vi "WLAN Configure SEM.vi"(0 "Instrument Handle In":refnum<k21>, 1 "Selector String":string, 5 "WLAN SEM Configuration":T1={"Sweep Time Auto"=1, "Sweep Time (s)"=0.001, "Span Auto"=1, "Span (Hz)"=100000000.0, "Averaging Enabled"=0, "Averaging Count"=5, "Averaging Type"=0} {"Averaging Type" items=["RMS", "Log", "Scalar", "Max", "Min"]; "Averaging Enabled" items=["False", "True"]; "Span (Hz)" format="%.3p"; "Span Auto" items=["False", "True"]; "Sweep Time (s)" format="%.3p"; "Sweep Time Auto" items=["False", "True"]}, 11 "error in (no error)":errorcluster) -> (4 "Instrument Handle Out":refnum<k21>, 15 "error out":errorcluster)   [LabVIEW 2016, in "RFmxWLAN.lvlib"]
uses:
  RFmxWLAN.lvlib
  Typedefs/WLAN SEM Configuration.ctl
  <resource>/objmgr/RFmxWLAN.rc
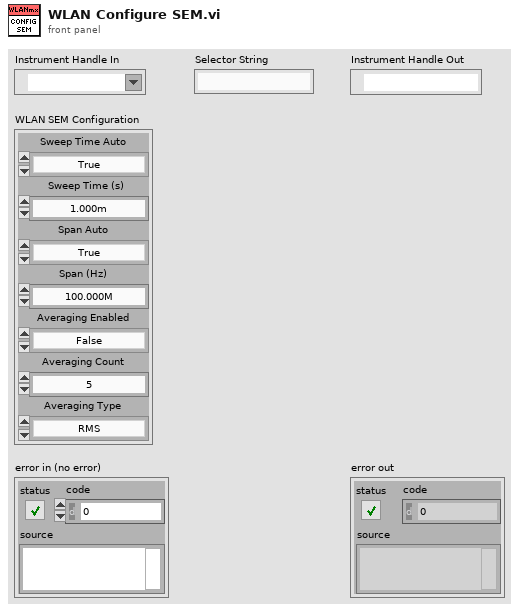
[diagram p1: front panel]
types:
  T1 = typedef "RFmxWLAN.lvlib/WLAN SEM Configuration.ctl" = cluster{"Sweep Time Auto":i32, "Sweep Time (s)":dbl, "Span Auto":i32, "Span (Hz)":dbl, "Averaging Enabled":i32, "Averaging Count":i32, "Averaging Type":i32}
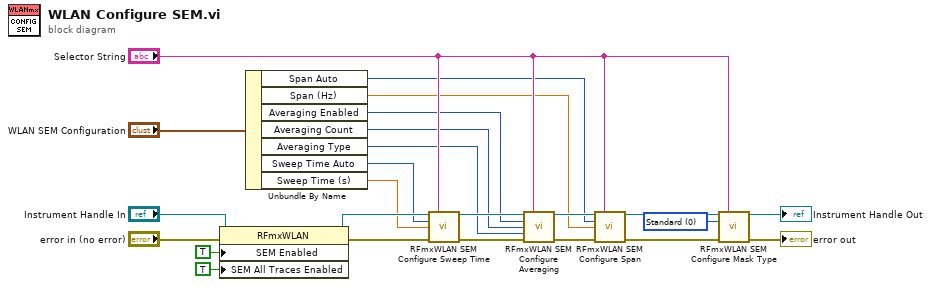
[diagram p0: block diagram]
diagram:
  w3 = 0 items=["Standard", "Custom"] ("Mask Type")
  n1 = property class="RFmxWLAN"(reference="Instrument Handle In", error in="error in (no error)", "SEM Enabled"=TRUE, "SEM All Traces Enabled"=TRUE) -> (reference out=w13:refnum<k21>, error out=w19:errorcluster)
  n2 = Unbundle By Name("WLAN SEM Configuration") -> ("Span Auto"=w2:i32, "Span (Hz)"=w1:dbl, "Averaging Enabled"=w4:i32, "Averaging Count"=w5:i32, "Averaging Type"=w6:i32, "Sweep Time Auto"=w8:i32, "Sweep Time (s)"=w7:dbl)
  n3 = call <vilib>:"RFmxWLAN SEM Configure Sweep Time.vi"("Instrument Handle In"=w13, "Selector String"="Selector String", "Sweep Time Auto"=w8, "Sweep Time Interval (s)"=w7, "error in (no error)"=w19) -> ("Instrument Handle Out"=w14:refnum<k21>, "error out"=w15:errorcluster)  [unwired: 9 in]
  n4 = call <vilib>:"RFmxWLAN SEM Configure Averaging.vi"("Instrument Handle In"=w14, "Selector String"="Selector String", "Averaging Enabled"=w4, "Averaging Count"=w5, "Averaging Type"=w6, "error in (no error)"=w15) -> ("Instrument Handle Out"=w11:refnum<k21>, "error out"=w20:errorcluster)  [unwired: 8 in]
  n5 = call <vilib>:"RFmxWLAN SEM Configure Span.vi"("Instrument Handle In"=w11, "Selector String"="Selector String", "Span Auto"=w2, "Span (Hz)"=w1, "error in (no error)"=w20) -> ("Instrument Handle Out"=w10:refnum<k21>, "error out"=w12:errorcluster)  [unwired: 9 in]
  n6 = call <vilib>:"RFmxWLAN SEM Configure Mask Type.vi"("Instrument Handle In"=w10, "Selector String"="Selector String", "Mask Type"=w3, "error in (no error)"=w12) -> ("Instrument Handle Out"=→"Instrument Handle Out":refnum<k21>, "error out"=→"error out":errorcluster)  [unwired: 10 in]
